vi "Splash Screen.vi"(8 "Error In":errorcluster) -> ()   [LabVIEW 2014]
uses:
  <vilib>/Ovak Technologies/Flat User Interface Controls Suite/Numeric/Horizontal Progress Bar.ctl
  SubVI/State/SubVI/Set Splash Screen State.vi
  SubVI/State/SubVI/Get Splash Screen State.vi
  <vilib>/Ovak Technologies/Flat User Interface Controls Suite/Flat User Interface Controls Suite.lvlib
panel:
  out "Horizontal Progress Bar":T1 scale=0.0..70.0
  out "Error Out":errorcluster
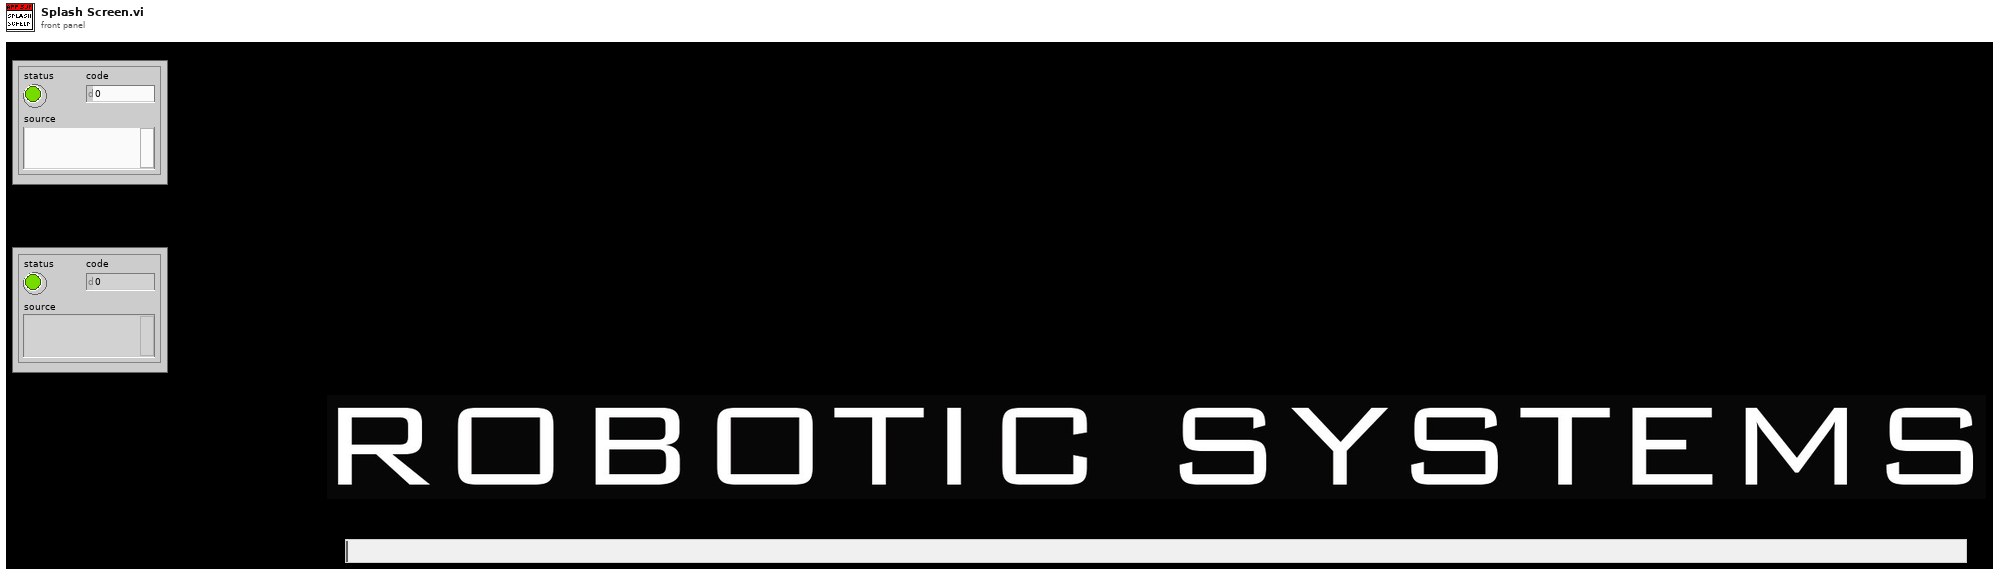
[diagram p1: front panel]
types:
  T1 = typedef "Flat User Interface Controls Suite.lvlib/Horizontal Progress Bar.ctl" = u8
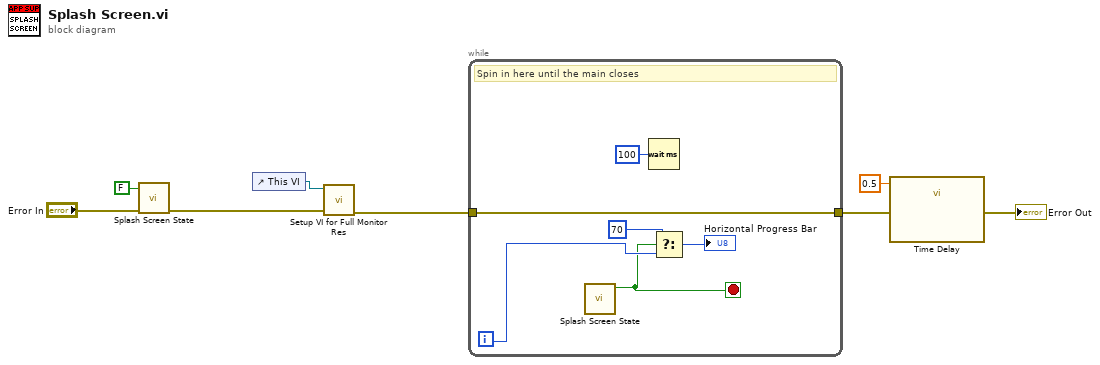
[diagram p0: block diagram]
diagram:
  n1 = call-poly "Splash Screen State.vi"("Error In"="Error In", "Close Splash Screen"=FALSE) -> ("Error Out"=w6:errorcluster)  [unwired: 9 in]
  n2 = control-ref of="This VI"() -> (w8:refnum<vi>)
  n3 = call "Setup VI for Full Monitor Res.vi"("Error In"=w6, "This VI"=w8) -> ("Error Out"=w7:errorcluster)  [unwired: 8 in, 1 out]
  n4 = while {
    tunnel: w7 -> [w13]
    tunnel: [w13] -> w3
    i -> [w12]
    stop <- w9 stop-if-true
    # "Spin in here until the main closes"
    n5 = call-poly "Splash Screen State.vi"() -> ("Close Splash Screen Out"=w9:bool)  [unwired: 10 in, 1 out]
    n6 = Wait (ms)(milliseconds to wait=u32 100) -> ()  [unwired: 1 out]
    n7 = Select(t=70, s=w9, f=w12) -> (s? t:f=→"Horizontal Progress Bar":i32)
  }
  n8 = call "Time Delay"("error in (no error)"=w3, "Delay Time (s)"=0.5) -> ("error out"=→"Error Out":errorcluster)  [unwired: 9 in]
